vi "Read Message Box.vi"(9 "RasPi Compiler in":refnum<class "RasPi Compiler.lvclass">) -> (3 "RasPi Compiler out":refnum<class "RasPi Compiler.lvclass">, 4 "Message Box":refnum<class "MessageBox.lvclass">)   [LabVIEW 2014, in "RasPi Compiler.lvclass"]
uses:
  RasPi Compiler.lvclass
  RasPi_Services/MessageBox/MessageBox.lvclass
  RasPi Compiler.lvclass/RasPi Compiler.ctl
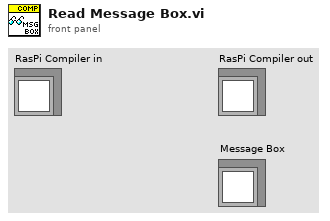
[diagram p1: front panel]
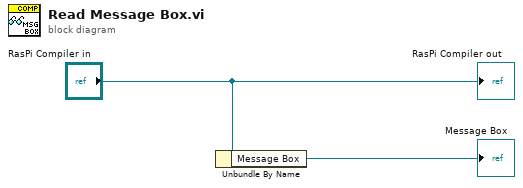
[diagram p0: block diagram]
diagram:
  n1 = Unbundle By Name("RasPi Compiler in") -> ("Message Box"=→"Message Box":refnum<class "MessageBox.lvclass">)
  "RasPi Compiler out" <- "RasPi Compiler in"
